vi "COD测量模式全局.vi"() -> ()   [LabVIEW 2016, in "斯坦道CODMn.lvlib"]
panel:
  out "测量模式文字实时":string
  out "CODMn工作状态":T1(ring)
  out "加标回收启动时间":timestamp format="%<%Y/%m/%d %H:%M:%S>T"
  out "水样启动时间":timestamp format="%<%Y/%m/%d %H:%M:%S>T"
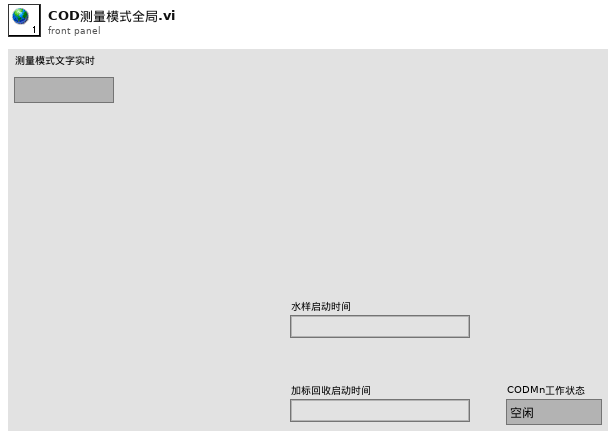
[diagram p1: front panel]
types:
  T1 = enum16{"空闲", "水样测试", "标样核查", "零点核查", "跨度核查", "空白测试", "平行样测试", "质控样", "空白校准", "标样校准", "加标回收"}
diagram:
